vi "test_F9P_232-2.vi"() -> ()   [LabVIEW 2019] (continued)
217,25,84,08,134,34,3*7E\r\n$GLGSV,2,2,06,85,63,113,24,86,52,337,,3*7F\r\n$GAGSV,3,1,09,02,04,287,05,04,68,084,40,09,44,196,42,11,78,040,40,7*7A\r\n$GAGSV,3,2,09,12,32,115,26,18,56,283,37,19,17,042,32,25,01,240,,7*76\r\n$GAGSV,3,3,09,36,35,314,37,7*4B\r\n$GAGSV,3,1,09,02,04,287,,04,68,084,36,09,44,196,34,11,78,040,33,2*7E\r\n$GAGSV,3,2,09,12,32,115,30,18,56,283,43,19,17,042,,25,01,240,,2*76\r\n$GAGSV,3,3,09,36,35,314,39,2*40\r\n$GBGSV,4,1,14,04,35,133,,05,09,257,,06,27,182,,07,09,201,,1*7C\r\n$GBGSV,4,2,14,08,65,355,43,09,07,194,,10,16,222,,11,37,142,25,1*78\r\n$GBGSV,4,3,14,13,50,315,41,14,76,037,44,16,24,185,30,28,59,310,44,1*7B\r\n$GBGSV,4,4,14,33,73,239,40,34,13,142,25,1*7E\r\n$GBGSV,4,1,14,04,35,133,,05,09,257,,06,27,182,,07,09,201,,3*7E\r\n$GBGSV,4,2,14,08,65,355,37,09,07,194,,10,16,222,,11,37,142,34,3*79\r\n$GBGSV,4,3,14,13,50,315,36,14,76,037,40,16,24,185,27,28,59,310,,3*7B\r\n$GBGSV,4,4,14,33,73,239,,34,13,142,,3*7F\r\n$GNGLL,3723.62908,N,12657.00861,E,064409.00,A,A*70\r\n$GNRMC,064410.00,A,3723.62923,N,12657.00951,E,2.574,77.08,250720,,,A,V*30\r\n$GNVTG,77.08,T,,M,2.574,N,4.766,K,A*1C\r\n$GNGGA,064410.00,3723.62923,N,12657.00951,E,1,12,0.64,38.4,M,18.5,M,,*74\r\n$GNGSA,A,3,17,19,06,12,05,02,09,,,,,,1.15,0.64,0.96,1*0C\r\n$GNGSA,A,3,85,70,71,72,,,,,,,,,1.15,0.64,0.96,2*03\r\n$GNGSA,A,3,36,19,11,04,09,12,,,,,,,1.15,0.64,0.96,3*08\r\n$GNGSA,A,3,28,11,14,13,33,08,34,,,,,,1.15,0.64,0.96,4*0E\r\n$GPGSV,4,1,13,02,66,335,46,04,08,037,21,05,48,262,40,06,58,077,46,1*6F\r\n$GPGSV,4,2,13,07,06,104,21,09,38,057,48,12,18,262,29,13,09,191,23,1*6F\r\n$GPGSV,4,3,13,17,18,158,22,19,37,162,33,25,11,293,18,29,07,323,35,1*65\r\n$GPGSV,4,4,13,30,01,133,,1*55\r\n$GPGSV,4,1,13,02,66,335,,04,08,037,21,05,48,262,34,06,58,077,37,6*6F\r\n$GPGSV,4,2,13,07,06,104,,09,38,057,40,12,18,262,19,13,09,191,,6*61\r\n$GPGSV,4,3,13,17,18,158,16,19,37,162,,25,11,293,16,29,07,323,,6*6D\r\n$GPGSV,4,4,13,30,01,133,,6*52\r\n$GLGSV,2,1,06,70,54,030,34,71,69,224,39,72,18,217,46,84,08,134,20,1*72\r\n$GLGSV,2,2,06,85,63,113,32,86,52,337,,1*7A\r\n$GLGSV,2,1,06,70,54,030,,71,69,224,28,72,18,217,25,84,08,134,30,3*73\r\n$GLGSV,2,2,06,85,63,113,31,86,52,337,,3*7B\r\n$GAGSV,3,1,09,02,04,287,08,04,68,084,39,09,44,196,41,11,78,040,38,7*75\r\n$GAGSV,3,2,09,12,32,115,31,18,56,283,39,19,17,042,27,25,01,240,,7*7A\r\n$GAGSV,3,3,09,36,35,314,34,7*48\r\n$GAGSV,3,1,09,02,04,287,,04,68,084,34,09,44,196,31,11,78,040,33,2*79\r\n$GAGSV,3,2,09,12,32,115,29,18,56,283,44,19,17,042,,25,01,240,,2*79\r\n$GAGSV,3,3,09,36,35,314,37,2*4E\r\n$GBGSV,4,1,14,04,35,133,,05,09,257,,06,27,182,,07,09,201,,1*7C\r\n$GBGSV,4,2,14,08,65,355,43,09,07,194,,10,16,222,,11,37,142,31,1*7D\r\n$GBGSV,4,3,14,13,50,315,42,14,76,037,42,16,24,185,30,28,59,310,43,1*79\r\n$GBGSV,4,4,14,33,73,239,41,34,13,142,25,1*7F\r\n$GBGSV,4,1,14,04,35,133,,05,09,257,,06,27,182,,07,09,201,,3*7E\r\n$GBGSV,4,2,14,08,65,355,36,09,07,194,,10,16,222,,11,37,142,30,3*7C\r\n$GBGSV,4,3,14,13,50,315,40,14,76,037,38,16,24,185,26,28,59,310,,3*74\r\n$GBGSV,4,4,14,33,73,239,,34,13,142,,3*7F\r\n$GNGLL,3723.62923,N,12657.00951,E,064410.00,A,A*73\r\n$GNRMC,064411.00,A,3723.62947,N,12657.01039,E,2.677,72.55,250720,,,A,V*38\r\n$GNVTG,72.55,T,,M,2.677,N,4.958,K,A*12\r\n$GNGGA,064411.00,3723.62947,N,12657.01039,E,1,12,0.64,38.2,M,18.5,M,,*77\r\n$GNGSA,A,3,17,19,06,12,05,02,09,,,,,,1.15,0.64,0.96,1*0C\r\n$GNGSA,A,3,85,70,71,72,,,,,,,,,1.15,0.64,0.96,2*03\r\n$GNGSA,A,3,36,19,11,04,09,12,,,,,,,1.15,0.64,0.96,3*08\r\n$GNGSA,A,3,28,11,14,13,33,08,34,,,,,,1.15,0.64,0.96,4*0E\r\n$GPGSV,4,1,13,02,66,335,46,04,08,037,21,05,48,262,40,06,58,077,44,1*6D\r\n$GPGSV,4,2,13,07,06,104,19,09,38,057,45,12,18,262,28,13,09,191,23,1*68\r\n$GPGSV,4,3,13,17,18,158,22,19,37,162,34,25,11,293,16,29,07,323,40,1*6E\r\n$GPGSV,4,4,13,30,01,133,,1*55\r\n$GPGSV,4,1,13,02,66,335,,04,08,037,20,05,48,262,34,06,58,077,36,6*6F\r\n$GPGSV,4,2,13,07,06,104,,09,38,057,41,12,18,262,19,13,09,191,,6*60\r\n$GPGSV,4,3,13,17,18,158,14,19,37,162,,25,11,293,15,29,07,323,,6*6C\r\n$GPGSV,4,4,13,30,01,133,,6*52\r\n$GLGSV,2,1,06,70,54,030,34,71,69,224,41,72,18,217,48,84,08,134,19,1*79\r\n$GLGSV,2,2,06,85,63,113,30,86,52,337,,1*78\r\n$GLGSV,2,1,06,70,54,030,,71,69,224,28,72,18,217,34,84,08,134,28,3*7A\r\n$GLGSV,2,2,06,85,63,113,30,86,52,337,,3*7A\r\n$GAGSV,3,1,09,02,04,287,10,04,68,084,41,09,44,196,40,11,78,040,40,7*7D\r\n$GAGSV,3,2,09,12,32,115,26,18,56,283,40,19,17,042,31,25,01,240,,7*75\r\n$GAGSV,3,3,09,36,35,314,32,7*4E\r\n$GAGSV,3,1,09,02,04,287,,04,68,084,37,09,44,196,34,11,78,040,32,2*7E\r\n$GAGSV,3,2,09,12,32,115,27,18,56,283,43,19,17,042,35,25,01,240,,2*76\r\n$GAGSV,3,3,09,36,35,314,37,2*4E\r\n$GBGSV,4,1,14,04,35,133,,05,09,257,,06,27,182,,07,09,201,,1*7C\r\n$GBGSV,4,2,14,08,65,355,43,09,07,194,,10,16,222,,11,37,142,26,1*7B\r\n$GBGSV,4,3,14,13,50,315,40,14,76,037,43,16,24,185,30,28,59,310,42,1*7B\r\n$GBGSV,4,4,14,33,73,239,41,34,13,142,25,1*7F\r\n$GBGSV,4,1,14,04,35,133,,05,09,257,,06,27,182,,07,09,201,,3*7E\r\n$GBGSV,4,2,14,08,65,355,35,09,07,194,,10,16,222,,11,37,142,36,3*79\r\n$GBGSV,4,3,14,13,50,315,36,14,76,037,37,16,24,185,24,28,59,310,,3*78\r\n$GBGSV,4,4,14,33,73,239,,34,13,142,,3*7F\r\n$GNGLL,3723.62947,N,12657.01039,E,064411.00,A,A*76\r\n$GNRMC,064412.00,A,3723.62972,N,12657.01126,E,2.612,69.92,250720,,,A,V*30\r\n$GNVTG,69.92,T,,M,2.612,N,4.838,K,A*17\r\n$GNGGA,064412.00,3723.62972,N,12657.01126,E,1,12,0.64,38.1,M,18.5,M,,*7E\r\n$GNGSA,A,3,17,19,06,12,05,02,09,,,,,,1.15,0.64,0.96,1*0C\r\n$GNGSA,A,3,85,70,71,72,,,,,,,,,1.15,0.64,0.96,2*03\r\n$GNGSA,A,3,36,19,11,04,09,12,,,,,,,1.15,0.64,0.96,3*08\r\n$GNGSA,A,3,28,11,14,13,33,08,34,,,,,,1.15,0.64,0.96,4*0E\r\n$GPGSV,4,1,13,02,66,335,44,04,08,037,,05,48,262,42,06,58,077,45,1*6F\r\n$GPGSV,4,2,13,07,06,104,,09,38,057,42,12,18,262,32,13,09,191,,1*6D\r\n$GPGSV,4,3,13,17,18,158,27,19,37,162,30,25,11,293,16,29,07,323,39,1*61\r\n$GPGSV,4,4,13,30,01,133,,1*55\r\n$GPGSV,4,1,13,02,66,335,,04,08,037,20,05,48,262,34,06,58,077,36,6*6F\r\n$GPGSV,4,2,13,07,06,104,,09,38,057,42,12,18,262,20,13,09,191,,6*69\r\n$GPGSV,4,3,13,17,18,158,13,19,37,162,,25,11,293,15,29,07,323,,6*6B\r\n$GPGSV,4,4,13,30,01,133,,6*52\r\n$GLGSV,2,1,06,70,54,030,34,71,69,224,41,72,18,217,48,84,08,134,18,1*78\r\n$GLGSV,2,2,06,85,63,113,35,86,52,337,,1*7D\r\n$GLGSV,2,1,06,70,54,030,,71,69,224,29,72,18,217,30,84,08,134,19,3*7D\r\n$GLGSV,2,2,06,85,63,113,29,86,52,337,,3*72\r\n$GAGSV,3,1,09,02,04,287,09,04,68,084,43,09,44,196,40,11,78,040,40,7*77\r\n$GAGSV,3,2,09,12,32,115,31,18,56,283,41,19,17,042,26,25,01,240,,7*74\r\n$GAGSV,3,3,09,36,35,314,40,7*4B\r\n$GAGSV,3,1,09,02,04,287,,04,68,084,39,09,44,196,32,11,78,040,32,2*76\r\n$GAGSV,3,2,09,12,32,115,27,18,56,283,43,19,17,042,,25,01,240,,2*70\r\n$GAGSV,3,3,09,36,35,314,39,2*40\r\n$GBGSV,4,1,14,04,35,133,,05,09,257,,06,27,182,,07,09,201,,1*7C\r\n$GBGSV,4,2,14,08,65,355,43,09,07,194,,10,16,222,,11,37,142,31,1*7D\r\n$GBGSV,4,3,14,13,50,315,35,14,76,037,44,16,24,185,29,28,59,310,44,1*70\r\n$GBGSV,4,4,14,33,73,239,42,34,13,142,30,1*78\r\n$GBGSV,4,1,14,04,35,133,,05,09,257,,06,27,182,,07,09,201,,3*7E\r\n$GBGSV,4,2,14,08,65,355,36,09,07,194,,10,16,222,,11,37,142,33,3*7F\r\n$GBGSV,4,3,14,13,50,315,29,14,76,037,39,16,24,185,23,28,59,310,,3*7F\r\n$GBGSV,4,4,14,33,73,239,,34,13,142,,3*7F\r\n$GNGLL,3723.62972,N,12657.01126,E,064412.00,A,A*7C\r\n$GNRMC,064413.00,A,3723.62994,N,12657.01207,E,2.382,70.38,250720,,,A,V*3D\r\n$GNVTG,70.38,T,,M,2.382,N,4.412,K,A*17\r\n$GNGGA,064413.00,3723.62994,N,12657.01207,E,1,12,0.64,38.3,M,18.5,M,,*75\r\n$GNGSA,A,3,17,19,06,12,05,02,09,,,,,,1.15,0.64,0.96,1*0C\r\n$GNGSA,A,3,85,70,71,72,,,,,,,,,1.15,0.64,0.96,2*03\r\n$GNGSA,A,3,36,19,11,04,09,12,,,,,,,1.15,0.64,0.96,3*08\r\n$GNGSA,A,3,28,11,14,13,33,08,,,,,,,1.15,0.64,0.96,4*09\r\n$GPGSV,4,1,13,02,66,335,42,04,08,037,19,05,48,262,39,06,58,077,47,1*6F\r\n$GPGSV,4,2,13,07,06,104,,09,38,057,40,12,18,262,28,13,09,191,,1*64\r\n$GPGSV,4,3,13,17,18,158,25,19,37,162,30,25,11,293,,29,07,323,34,1*69\r\n$GPGSV,4,4,13,30,01,133,,1*55\r\n$GPGSV,4,1,13,02,66,335,,04,08,037,20,05,48,262,35,06,58,077,39,6*61\r\n$GPGSV,4,2,13,07,06,104,,09,38,057,39,12,18,262,18,13,09,191,,6*6E\r\n$GPGSV,4,3,13,17,18,158,13,19,37,162,,25,11,293,16,29,07,323,,6*68\r\n$GPGSV,4,4,13,30,01,133,,6*52\r\n$GLGSV,2,1,06,70,54,030,27,71,69,224,42,72,18,217,41,84,08,134,17,1*7F\r\n$GLGSV,2,2,06,85,63,113,36,86,52,337,,1*7E\r\n$GLGSV,2,1,06,70,54,030,,71,69,224,29,72,18,217,34,84,08,134,28,3*7B\r\n$GLGSV,2,2,06,85,63,113,28,86,52,337,,3*73\r\n$GAGSV,3,1,09,02,04,287,09,04,68,084,45,09,44,196,37,11,78,040,40,7*71\r\n$GAGSV,3,2,09,12,32,115,32,18,56,283,43,19,17,042,25,25,01,240,,7*76\r\n$GAGSV,3,3,09,36,35,314,41,7*4A\r\n$GAGSV,3,1,09,02,04,287,,04,68,084,37,09,44,196,34,11,78,040,32,2*7E\r\n$GAGSV,3,2,09,12,32,115,28,18,56,283,45,19,17,042,30,25,01,240,,2*7A\r\n$GAGSV,3,3,09,36,35,314,39,2*40\r\n$GBGSV,4,1,14,04,35,133,,05,09,257,,06,27,182,,07,09,201,,1*7C\r\n$GBGSV,4,2,14,08,65,355,43,09,07,194,,10,16,222,,11,37,142,31,1*7D\r\n$GBGSV,4,3,14,13,50,315,39,14,76,037,43,16,24,185,21,28,59,310,44,1*73\r\n$GBGSV,4,4,14,33,73,239,43,34,13,142,,1*7A\r\n$GBGSV,4,1,14,04,35,133,,05,09,257,,06,27,182,,07,09,201,,3*7E\r\n$GBGSV,4,2,14,08,65,355,37,09,07,194,,10,16,222,,11,37,142,30,3*7D\r\n$GBGSV,4,3,14,13,50,315,34,14,76,037,39,16,24,185,22,28,59,310,,3*72\r\n$GBGSV,4,4,14,33,73,239,,34,13,142,,3*7F\r\n$GNGLL,3723.62994,N,12657.01207,E,064413.00,A,A*75\r\n$GNRMC,064414.00,A,3723.63019,N,12657.01291,E,2.603,69.89,250720,,,A,V*36\r\n$GNVTG,69.89,T,,M,2.603,N,4.821,K,A*15\r\n$GNGGA,064414.00,3723.63019,N,12657.01291,E,1,12,0.64,38.4,M,18.5,M,,*77\r\n$GNGSA,A,3,17,19,06,12,05,02,09,,,,,,1.15,0.64,0.96,1*0C\r\n$GNGSA,A,3,85,70,71,72,,,,,,,,,1.15,0.64,0.96,2*03\r\n$GNGSA,A,3,36,19,11,04,09,12,,,,,,,1.15,0.64,0.96,3*08\r\n$GNGSA,A,3,28,11,14,13,33,08,,,,,,,1.15,0.64,0.96,4*09\r\n$GPGSV,4,1,13,02,66,335,43,04,08,037,19,05,48,262,32,06,58,077,47,1*65\r\n$GPGSV,4,2,13,07,06,104,23,09,38,057,40,12,18,262,26,13,09,191,27,1*6E\r\n$GPGSV,4,3,13,17,18,158,26,19,37,162,30,25,11,293,26,29,07,323,30,1*6A\r\n$GPGSV,4,4,13,30,01,133,,1*55\r\n$GPGSV,4,1,13,02,66,335,,04,08,037,21,05,48,262,38,06,58,077,37,6*63\r\n$GPGSV,4,2,13,07,06,104,,09,38,057,42,12,18,262,17,13,09,191,,6*6D\r\n$GPGSV,4,3,13,17,18,158,,19,37,162,,25,11,293,15,29,07,323,,6*69\r\n$GPGSV,4,4,13,30,01,133,,6*52\r\n$GLGSV,2,1,06,70,54,030,21,71,69,224,42,72,18,217,39,84,08,134,17,1*76\r\n$GLGSV,2,2,06,85,63,113,35,86,52,337,,1*7D\r\n$GLGSV,2,1,06,70,54,030,,71,69,224,29,72,18,217,30,84,08,134,22,3*75\r\n$GLGSV,2,2,06,85,63,113,28,86,52,337,,3*73\r\n$GAGSV,3,1,09,02,04,287,07,04,68,084,45,09,44,196,41,11,78,040,40,7*7E\r\n$GAGSV,3,2,09,12,32,115,27,18,56,283,42,19,17,042,31,25,01,240,,7*76\r\n$GAGSV,3,3,09,36,35,314,40,7*4B\r\n$GAGSV,3,1,09,02,04,287,,04,68,084,34,09,44,196,37,11,78,040,32,2*7E\r\n$GAGSV,3,2,09,12,32,115,28,18,56,283,43,19,17,042,,25,01,240,,2*7F\r\n$GAGSV,3,3,09,36,35,314,41,2*4F\r\n$GBGSV,4,1,14,04,35,133,,05,09,257,,06,27,182,,07,09,201,,1*7C\r\n$GBGSV,4,2,14,08,65,355,41,09,07,194,,10,16,222,,11,37,142,31,1*7F\r\n$GBGSV,4,3,14,13,50,315,41,14,76,037,46,16,24,185,23,28,59,310,43,1*7C\r\n$GBGSV,4,4,14,33,73,239,42,34,13,142,,1*7B\r\n$GBGSV,4,1,14,04,35,133,,05,09,257,,06,27,182,,07,09,201,,3*7E\r\n$GBGSV,4,2,14,08,65,355,39,09,07,194,,10,16,222,,11,37,142,35,3*76\r\n$GBGSV,4,3,14,13,50,315,36,14,76,037,35,16,24,185,22,28,59,310,,3*7C\r\n$GBGSV,4,4,14,33,73,239,,34,13,142,,3*7F\r\n$GNGLL,3723.63019,N,12657.01291,E,064414.00,A,A*70\r\n$GNRMC,064415.00,A,3723.63048,N,12657.01379,E,2.743,67.58,250720,,,A,V*33\r\n$GNVTG,67.58,T,,M,2.743,N,5.080,K,A*10\r\n$GNGGA,064415.00,3723.63048,N,12657.01379,E,1,12,0.64,38.5,M,18.5,M,,*74\r\n$GNGSA,A,3,17,19,06,12,05,02,09,,,,,,1.15,0.64,0.96,1*0C\r\n$GNGSA,A,3,85,70,71,72,,,,,,,,,1.15,0.64,0.96,2*03\r\n$GNGSA,A,3,36,19,11,04,09,12,,,,,,,1.15,0.64,0.96,3*08\r\n$GNGSA,A,3,28,11,14,13,33,08,,,,,,,1.15,0.64,0.96,4*09\r\n$GPGSV,4,1,13,02,66,335,42,04,08,037,,05,48,262,38,06,58,077,46,1*67\r\n$GPGSV,4,2,13,07,06,104,23,09,38,057,40,12,18,262,,13,09,191,25,1*68\r\n$GPGSV,4,3,13,17,18,158,27,19,37,162,30,25,11,293,26,29,07,323,34,1*6F\r\n$GPGSV,4,4,13,30,01,133,,1*55\r\n$GPGSV,4,1,13,02,66,335,,04,08,037,21,05,48,262,39,06,58,077,37,6*62\r\n$GPGSV,4,2,13,07,06,104,,09,38,057,41,12,18,262,18,13,09,191,,6*61\r\n$GPGSV,4,3,13,17,18,158,,19,37,162,,25,11,293,15,29,07,323,,6*69\r\n$GPGSV,4,4,13,30,01,133,,6*52\r\n$GLGSV,2,1,06,70,54,030,34,71,69,224,41,72,18,217,43,84,08,134,16,1*7D\r\n$GLGSV,2,2,06,85,63,113,38,86,52,337,,1*70\r\n$GLGSV,2,1,06,70,54,030,,71,69,224,29,72,18,217,30,84,08,134,24,3*73\r\n$GLGSV,2,2,06,85,63,113,33,86,52,337,,3*79\r\n$GAGSV,3,1,09,02,04,287,10,04,68,084,43,09,44,196,41,11,78,040,40,7*7E\r\n$GAGSV,3,2,09,12,32,115,32,18,56,283,38,19,17,042,27,25,01,240,,7*78\r\n$GAGSV,3,3,09,36,35,314,38,7*44\r\n$GAGSV,3,1,09,02,04,287,,04,68,084,39,09,44,196,31,11,78,040,33,2*74\r\n$GAGSV,3,2,09,12,32,115,28,18,56,283,43,19,17,042,34,25,01,240,,2*78\r\n$GAGSV,3,3,09,36,35,314,40,2*4E\r\n$GBGSV,4,1,14,04,35,133,,05,09,257,,06,27,182,,07,09,201,,1*7C\r\n$GBGSV,4,2,14,08,65,355,41,09,07,194,,10,16,222,,11,37,142,30,1*7E\r\n$GBGSV,4,3,14,13,50,315,37,14,76,037,43,16,24,185,23,28,59,310,42,1*79\r\n$GBGSV,4,4,14,33,73,239,42,34,13,142,,1*7B\r\n$GBGSV,4,1,14,04,35,133,,05,09,257,,06,27,182,,07,09,201,,3*7E\r\n$GBGSV,4,2,14,08,65,355,31,09,07,194,,10,16,222,,11,37,142,33,3*78\r\n$GBGSV,4,3,14,13,50,315,37,14,76,037,33,16,24,185,22,28,59,310,,3*7B\r\n$GBGSV,4,4,14,33,73,239,,34,13,142,,3*7F\r\n$GNGLL,3723.63048,N,12657.01379,E,064415.00,A,A*72\r\n$GNRMC,064416.00,A,3723.63080,N,12657.01467,E,2.766,65.42,250720,,,A,V*32\r\n$GNVTG,65.42,T,,M,2.766,N,5.123,K,A*16\r\n$GNGGA,064416.00,3723.63080,N,12657.01467,E,1,12,0.64,38.5,M,18.5,M,,*7B\r\n$GNGSA,A,3,19,06,12,05,02,09,,,,,,,1.15,0.64,0.96,1*0A\r\n$GNGSA,A,3,85,70,71,72,,,,,,,,,1.15,0.64,0.96,2*03\r\n$GNGSA,A,3,36,19,11,04,09,12,,,,,,,1.15,0.64,0.96,3*08\r\n$GNGSA,A,3,28,11,14,13,33,08,,,,,,,1.15,0.64,0.96,4*09\r\n$GPGSV,4,1,13,02,66,335,40,04,08,037,18,05,48,262,37,06,58,077,48,1*6D\r\n$GPGSV,4,2,13,07,06,104,22,09,38,057,39,12,18,262,27,13,09,191,24,1*63\r\n$GPGSV,4,3,13,17,18,158,,19,37,162,28,25,11,293,25,29,07,323,29,1*6C\r\n$GPGSV,4,4,13,30,01,133,,1*55\r\n$GPGSV,4,1,13,02,66,335,,04,08,037,19,05,48,262,33,06,58,077,37,6*63\r\n$GPGSV,4,2,13,07,06,104,,09,38,057,40,12,18,262,18,13,09,191,,6*60\r\n$GPGSV,4,3,13,17,18,158,,19,37,162,,25,11,293,15,29,07,323,,6*69\r\n$GPGSV,4,4,13,30,01,133,,6*52\r\n$GLGSV,2,1,06,70,54,030,29,71,69,224,39,72,18,217,39,84,08,134,16,1*73\r\n$GLGSV,2,2,06,85,63,113,42,86,52,337,,1*7D\r\n$GLGSV,2,1,06,70,54,030,,71,69,224,28,72,18,217,23,84,08,134,23,3*77\r\n$GLGSV,2,2,06,85,63,113,27,86,52,337,,3*7C\r\n$GAGSV,3,1,09,02,04,287,08,04,68,084,44,09,44,196,41,11,78,040,38,7*7F\r\n$GAGSV,3,2,09,12,32,115,33,18,56,283,39,19,17,042,35,25,01,240,,7*7B\r\n$GAGSV,3,3,09,36,35,314,37,7*4B\r\n$GAGSV,3,1,09,02,04,287,,04,68,084,39,09,44,196,38,11,78,040,31,2*7F\r\n$GAGSV,3,2,09,12,32,115,32,18,56,283,43,19,17,042,31,25,01,240,,2*76\r\n$GAGSV,3,3,09,36,35,314,39,2*40\r\n$GBGSV,4,1,14,04,35,133,,05,09,257,,06,27,182,,07,09,201,,1*7C\r\n$GBGSV,4,2,14,08,65,355,39,09,07,194,,10,16,222,,11,37,142,29,1*79\r\n$GBGSV,4,3,14,13,50,315,32,14,76,037,45,16,24,185,24,28,59,310,40,1*7F\r\n$GBGSV,4,4,14,33,73,239,38,34,13,142,,1*76\r\n$GBGSV,4,1,14,04,35,133,,05,09,257,,06,27,182,,07,09,201,,3*7E\r\n$GBGSV,4,2,14,08,65,355,32,09,07,194,,10,16,222,,11,37,142,28,3*71\r\n$GBGSV,4,3,14,13,50,315,36,14,76,037,37,16,24,185,21,28,59,310,,3*7D\r\n$GBGSV,4,4,14,33,73,239,,34,13,142,,3*7F\r\n$GNGLL,3723.63080,N,12657.01467,E,064416.00,A,A*7D\r\n$GNRMC,064417.00,A,3723.63108,N,12657.01557,E,2.757,66.77,250720,,,A,V*37\r\n$GNVTG,66.77,T,,M,2.757,N,5.106,K,A*16\r\n$GNGGA,064417.00,3723.63108,N,12657.01557,E,1,12,0.62,38.6,M,18.5,M,,*7C\r\n$GNGSA,A,3,19,06,12,05,02,09,,,,,,,1.10,0.62,0.91,1*0E\r\n$GNGSA,A,3,85,70,71,72,,,,,,,,,1.10,0.62,0.91,2*07\r\n$GNGSA,A,3,36,19,11,04,09,12,,,,,,,1.10,0.62,0.91,3*0C\r\n$GNGSA,A,3,28,10,11,14,13,33,08,,,,,,1.10,0.62,0.91,4*0C\r\n$GPGSV,4,1,13,02,66,335,40,04,08,037,,05,48,262,36,06,58,077,48,1*65\r\n$GPGSV,4,2,13,07,06,104,22,09,38,057,34,12,18,262,26,13,09,191,22,1*69\r\n$GPGSV,4,3,13,17,18,158,23,19,37,162,28,25,11,293,26,29,07,323,29,1*6E\r\n$GPGSV,4,4,13,30,01,133,,1*55\r\n$GPGSV,4,1,13,02,66,335,,04,08,037,22,05,48,262,33,06,58,077,39,6*65\r\n$GPGSV,4,2,13,07,06,104,,09,38,057,39,12,18,262,18,13,09,191,,6*6E\r\n$GPGSV,4,3,13,17,18,158,,19,37,162,,25,11,293,18,29,07,323,,6*64\r\n$GPGSV,4,4,13,30,01,133,,6*52\r\n$GLGSV,2,1,06,70,54,030,32,71,69,224,39,72,18,217,41,84,08,134,15,1*75\r\n$GLGSV,2,2,06,85,63,113,39,86,52,337,,1*71\r\n$GLGSV,2,1,06,70,54,030,,71,69,224,26,72,18,217,26,84,08,134,22,3*7D\r\n$GLGSV,2,2,06,85,63,113,27,86,52,337,,3*7C\r\n$GAGSV,3,1,09,02,04,287,07,04,68,084,42,09,44,196,42,11,78,040,40,7*7A\r\n$GAGSV,3,2,09,12,32,115,32,18,56,283,36,19,17,042,31,25,01,240,,7*71\r\n$GAGSV,3,3,09,36,35,314,30,7*4C\r\n$GAGSV,3,1,09,02,04,287,,04,68,084,39,09,44,196,35,11,78,040,32,2*71\r\n$GAGSV,3,2,09,12,32,115,29,18,56,283,39,19,17,042,,25,01,240,,2*73\r\n$GAGSV,3,3,09,36,35,314,32,2*4B\r\n$GBGSV,4,1,14,04,35,133,,05,09,257,,06,27,182,,07,09,201,,1*7C\r\n$GBGSV,4,2,14,08,65,355,40,09,07,194,,10,16,222,33,11,37,142,31,1*7E\r\n$GBGSV,4,3,14,13,50,315,28,14,76,037,45,16,24,185,23,28,59,310,36,1*72\r\n$GBGSV,4,4,14,33,73,239,40,34,13,142,,1*79\r\n$GBGSV,4,1,14,04,35,133,,05,09,257,,06,27,182,,07,09,201,,3*7E\r\n$GBGSV,4,2,14,08,65,355,38,09,07,194,,10,16,222,,11,37,142,35,3*77\r\n$GBGSV,4,3,14,13,50,315,32,14,76,037,41,16,24,185,22,28,59,310,,3*7B\r\n$GBGSV,4,4,14,33,73,239,,34,13,142,,3*7F\r\n$GNGLL,3723.63108,N,12657.01557,E,064417.00,A,A*7F\r\n$GNRMC,064418.00,A,3723.63139,N,12657.01643,E,2.693,64.49,250720,,,A,V*3A\r\n$GNVTG,64.49,T,,M,2.693,N,4.988,K,A*1F\r\n$GNGGA,064418.00,3723.63139,N,12657.01643,E,1,12,0.62,38.6,M,18.5,M,,*77\r\n$GNGSA,A,3,19,06,12,05,02,09,,,,,,,1.10,0.62,0.91,1*0E\r\n$GNGSA,A,3,85,70,71,72,,,,,,,,,1.10,0.62,0.91,2*07\r\n$GNGSA,A,3,36,19,11,04,09,12,,,,,,,1.10,0.62,0.91,3*0C\r\n$GNGSA,A,3,28,10,11,14,13,33,08,,,,,,1.10,0.62,0.91,4*0C\r\n$GPGSV,4,1,13,02,66,335,41,04,08,037,25,05,48,262,38,06,58,077,48,1*6D\r\n$GPGSV,4,2,13,07,06,104,22,09,38,057,40,12,18,262,31,13,09,191,21,1*6F\r\n$GPGSV,4,3,13,17,18,158,24,19,37,162,32,25,11,293,26,29,07,323,28,1*63\r\n$GPGSV,4,4,13,30,01,133,,1*55\r\n$GPGSV,4,1,13,02,66,335,,04,08,037,23,05,48,262,36,06,58,077,39,6*61\r\n$GPGSV,4,2,13,07,06,104,,09,38,057,40,12,18,262,17,13,09,191,,6*6F\r\n$GPGSV,4,3,13,17,18,158,,19,37,162,,25,11,293,19,29,07,323,,6*65\r\n$GPGSV,4,4,13,30,01,133,,6*52\r\n$GLGSV,2,1,06,70,54,030,32,71,69,224,41,72,18,217,43,84,08,134,16,1*7B\r\n$GLGSV,2,2,06,85,63,113,36,86,52,337,,1*7E\r\n$GLGSV,2,1,06,70,54,030,,71,69,224,26,72,18,217,28,84,08,134,21,3*70\r\n$GLGSV,2,2,06,85,63,113,29,86,52,337,,3*72\r\n$GAGSV,3,1,09,02,04,287,10,04,68,084,42,09,44,196,40,11,78,040,40,7*7E\r\n$GAGSV,3,2,09,12,32,115,32,18,56,283,33,19,17,042,26,25,01,240,,7*72\r\n$GAGSV,3,3,09,36,35,314,33,7*4F\r\n$GAGSV,3,1,09,02,04,287,,04,68,084,39,09,44,196,35,11,78,040,32,2*71\r\n$GAGSV,3,2,09,12,32,115,,18,56,283,38,19,17,042,32,25,01,240,,2*78\r\n$GAGSV,3,3,09,36,35,314,37,2*4E\r\n$GBGSV,4,1,14,04,35,133,,05,09,257,,06,27,182,,07,09,201,,1*7C\r\n$GBGSV,4,2,14,08,65,355,39,09,07,194,,10,16,222,32,11,37,142,34,1*74\r\n$GBGSV,4,3,14,13,50,315,36,14,76,037,44,16,24,185,23,28,59,310,38,1*72\r\n$GBGSV,4,4,14,33,73,239,43,34,13,142,,1*7A\r\n$GBGSV,4,1,14,04,35,133,,05,09,257,,06,27,182,,07,09,201,,3*7E\r\n$GBGSV,4,2,14,08,65,355,35,09,07,194,,10,16,222,,11,37,142,32,3*7D\r\n$GBGSV,4,3,14,13,50,315,32,14,76,037,40,16,24,185,21,28,59,310,,3*79\r\n$GBGSV,4,4,14,33,73,239,,34,13,142,,3*7F\r\n$GNGLL,3723.63139,N,12657.01643,E,064418.00,A,A*74\r\n$GNRMC,064419.00,A,3723.63178,N,12657.01724,E,2.627,60.88,250720,,,A,V*38\r\n$GNVTG,60.88,T,,M,2.627,N,4.866,K,A*18\r\n$GNGGA,064419.00,3723.63178,N,12657.01724,E,1,12,0.62,38.4,M,18.5,M,,*71\r\n$GNGSA,A,3,19,06,12,05,02,17,09,,,,,,1.10,0.62,0.91,1*08\r\n$GNGSA,A,3
